vi "read_attributes.vi"(8 "error in (no error)":errorcluster, 11 "LatentDirichletAllocation in":refnum<class "LatentDirichletAllocation.lvclass">) -> (0 "error out":errorcluster, 2 "attributes":T1, 3 "LatentDirichletAllocation out":refnum<class "LatentDirichletAllocation.lvclass">)   [LabVIEW 2020, in "LatentDirichletAllocation.lvclass"]
uses:
  LatentDirichletAllocation.lvclass
  Controls/latent_dirichlet_allocation_attributes.ctl
  LatentDirichletAllocation.lvclass/LatentDirichletAllocation.ctl
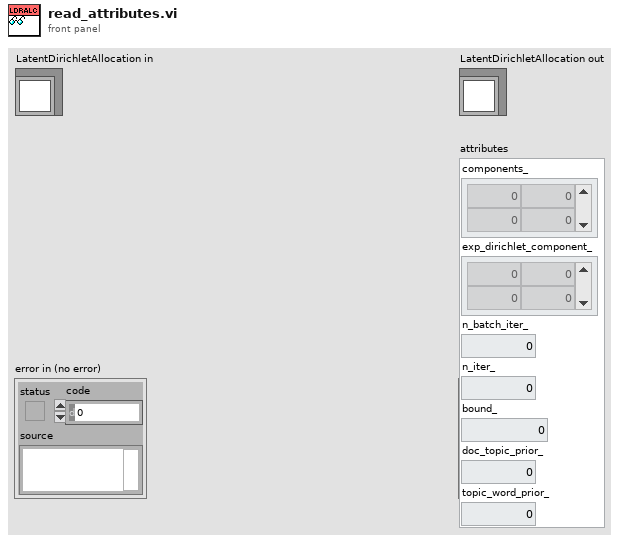
[diagram p1: front panel]
types:
  T1 = typedef "latent_dirichlet_allocation_attributes.ctl" = cluster{"components_":dbl[][], "exp_dirichlet_component_":dbl[][], "n_batch_iter_":dbl, "n_iter_":dbl, "bound_":dbl, "doc_topic_prior_":dbl, "topic_word_prior_":dbl}
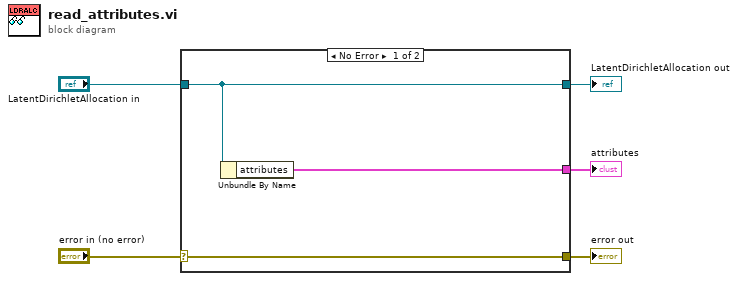
[diagram p0: block diagram]
diagram:
  n1 = case shown="No Error" "error in (no error)" {
    selector: "error in (no error)" -> [w8 w9]
    tunnel: [w8 w9] -> w4
    tunnel: [w7 w10] -> w2
    tunnel: "LatentDirichletAllocation in" -> [w7 w10]
    tunnel: [w6 _] -> w1
    frame No Error {
      n2 = Unbundle By Name(w7) -> ("attributes"=w6:T1)
    }
    frame Error {
    }
  }
  "error out" <- w4
  "LatentDirichletAllocation out" <- w2
  "attributes" <- w1
